vi "VI Tester UI.vi"() -> ()   [LabVIEW 2014, in "VI Tester Node.lvclass"]
uses:
  VI Tester Node.lvclass
  <vilib>/ni/Configuration Framework/Node/NodeRef.ctl
  <vilib>/ni/Configuration Framework/Node/NISE_CEF_Node.lvclass
  <vilib>/ni/AMC/Message Queue.ctl
  <vilib>/ni/AMC/Message.ctl
  <vilib>/ni/Tools/Keyed Array/KeyedArray.ctl
  <vilib>/ni/Configuration Framework/Node/UserEventRef.ctl
  <vilib>/ni/Configuration Framework/Controls/EventCluster.ctl
  VI Tester Node.lvclass/VI Tester Node.ctl
  Classes/Build Job/Build Job.lvclass/Build Job.ctl
  <vilib>/ni/AMC/Create Single Message.vi
  <vilib>/ni/AMC/Update Message Routing Info.vi
  <vilib>/ni/AMC/Send Message.vi
  <vilib>/ni/AMC/AMC.lvlib
  Classes/Build Job/Build Job.lvclass
  <vilib>/ni/Tools/Keyed Array/Tools_KeyedArray.lvlib
  <vilib>/ni/Configuration Framework/NISE_CEF_TreeControl.lvlib
panel:
  in  "Test Suite":path=path "C:/Projects/LabVIEW Continuous Integration/LabVIEW Continuous Integration.lvproj"
  in  "Description":string
  in  "user event":T1
  in  "main queue":T2
  in  "node ref":T3
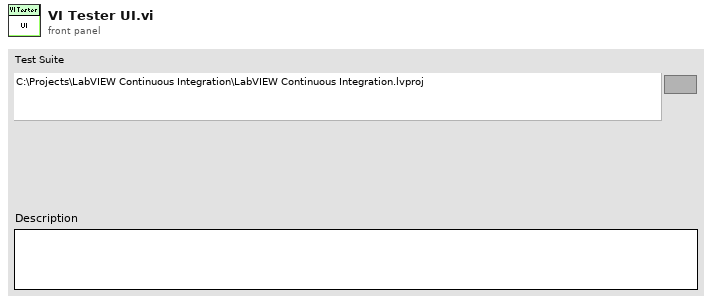
[diagram p1: front panel]
types:
  T1 = typedef "NISE_CEF_Node.lvclass/UserEventRef.ctl" = refnum<user-event>
  T2 = typedef "AMC.lvlib/Message Queue.ctl" = refnum<queue>
  T3 = typedef "NISE_CEF_Node.lvclass/NodeRef.ctl" = refnum<data-value>
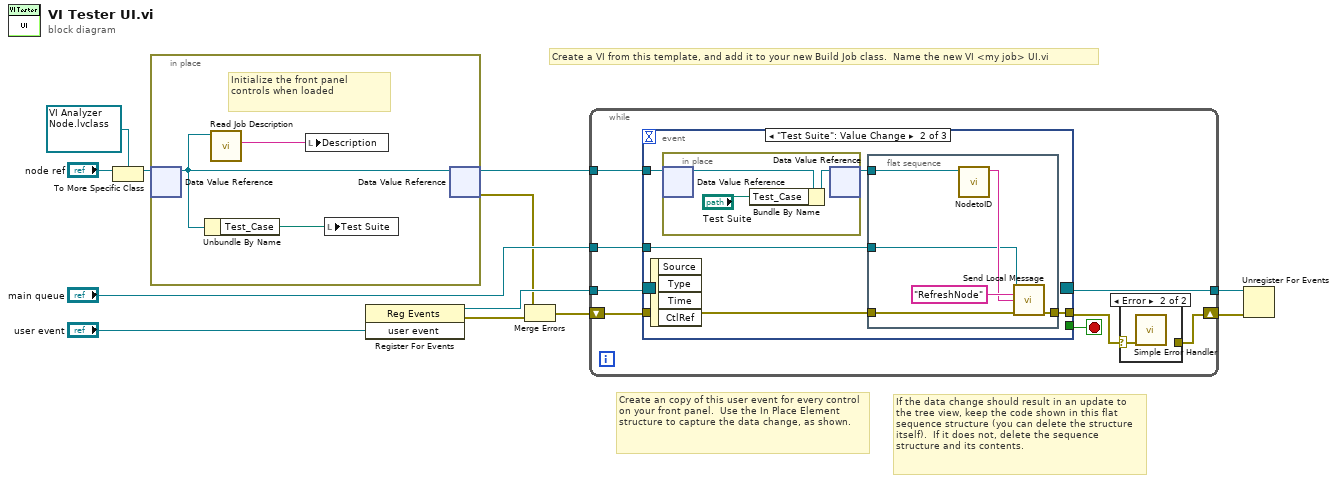
[diagram p0: block diagram]
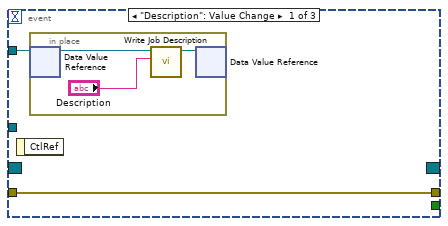
[diagram p3: hidden frame]
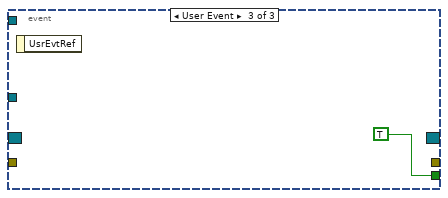
[diagram p4: hidden frame]
diagram:
  # "Create a VI from this template, and add it to your new Build Job class.  Name the new VI <my job> UI.vi"
  # "If the data change should result in an update to the tree view, keep the code shown in this flat sequence structure (you can delete the structure itself).  If it does not, delete the sequence structure and its contents."
  # "Create an copy of this user event for every control on your front panel.  Use the In Place Element structure to capture the data change, as shown."
  n1 = To More Specific Class(target class=refnum<data-value> refnum ("data value reference"), reference="node ref") -> (specific class reference=w6:refnum<data-value>)  [unwired: 1 in, 1 out]
  n2 = in-place {
    # "Initialize the front panel controls when loaded"
    n3 = in-place-dvr #1(w6) -> (w14:refnum<class "VI Tester Node.lvclass">)  [unwired: 1 out]
    n4 = Unbundle By Name(w14) -> ("Test_Case"=w13:path)
    n5 = call-dynamic "Read Job Description.vi"("Build Job in"=w14) -> ("Job Description"=w15:string)  [unwired: 10 in]
    n6 = local write "Description"(w15) -> ()
    n7 = local write "Test Suite"(w13) -> ()
    n8 = in-place-dvr #1(w14) -> (w2:refnum<data-value>, w4:errorcluster)
  }
  n9 = register-events("user event") -> (reference out=w10:refnum<event-registration>, error out=w5:errorcluster)  [unwired: 2 in]
  n10 = Merge Errors(w4, w5) -> (w3:errorcluster)
  n11 = while {
    tunnel: w2 -> [w23]
    tunnel: "main queue" -> [w22]
    tunnel: w10 -> [w21]
    tunnel: [w20] -> w9
    shift-right: [w16] -> w8
    shift-left: w3 -> [w19]
    stop <- w18 stop-if-true
    n12 = event shown="[1] \"Test Suite\": Value Change" {
      selector: w21 -> [_ _ _]
      dyn-events: [_ _ _] -> w20
      timeout: _ -> [_ _ _]
      tunnel: w23 -> [w27 w35 _]
      tunnel: w22 -> [_ w31 _]
      tunnel: [_ _ TRUE] -> w18
      tunnel: [w26 w32 _] -> w17
      tunnel: w19 -> [w26 w33 _]
      event "Description": Value Change {
        n13 = event-data() -> ()  [unwired: 1 in, 1 out]
        n14 = in-place {
          n15 = in-place-dvr #2(w27) -> (w30:refnum<class "VI Tester Node.lvclass">)  [unwired: 1 out]
          n16 = call "Write Job Description.vi"("Job Description"="Description", "Build Job in"=w30) -> ("Build Job out"=w29:refnum<class "VI Tester Node.lvclass">)  [unwired: 9 in]
          n17 = in-place-dvr #2(w29) -> ()  [unwired: 2 out]
        }
      }
      event "Test Suite": Value Change {
        n18 = event-data() -> ()  [unwired: 1 in, 4 out]
        n19 = in-place {
          n20 = in-place-dvr #3(w35) -> (w44:refnum<class "VI Tester Node.lvclass">)  [unwired: 1 out]
          n21 = Bundle By Name(cluster=w44, "Test_Case"="Test Suite") -> (w43:refnum<class "VI Tester Node.lvclass">)
          n22 = in-place-dvr #3(w43) -> (w34:refnum<data-value>)  [unwired: 1 out]
        }
        n23 = flat-sequence {
          tunnel: w34 -> [w39]
          tunnel: w33 -> [w38]
          tunnel: [w37] -> w32
          tunnel: w31 -> [w36]
          frame #0 {
            n24 = call <vilib>:"NodetoID.vi"("node ref"=w39) -> ("ID"=w40:string)  [unwired: 9 in, 1 out]
            n25 = call <vilib>:"Send Local Message.vi"("message queue in"=w36, "message name"="RefreshNode" ("Message Name"), "message value"=w40, "error in"=w38) -> ("error out"=w37:errorcluster)  [unwired: 9 in, 2 out]
          }
        }
      }
      event User Event {
        n26 = event-data() -> ()  [unwired: 1 in, 1 out]
      }
    }
    n27 = case shown="Error" w17 {
      selector: w17 -> [w24 w25]
      tunnel: [w24 _] -> w16
      frame No Error {
      }
      frame Error {
        n28 = call <vilib>:"Simple Error Handler.vi"("error in (no error)"=w25) -> ()  [unwired: 4 in, 5 out]
      }
    }
  }
  n29 = Unregister For Events(event registration refnum=w9, error in=w8) -> ()  [unwired: 1 out]
